vi "mean_Scope.vi"(0 "instrument handle in":refnum<k15>, 5 "pulses":i32, 7 "channels":string="0", 9 "record length":i32, 11 "error in":errorcluster) -> (4 "instrument handle out":refnum<k15>, 6 "signal out":dbl[](array[numeric]), 8 "dt":dbl, 15 "error out":errorcluster)   [LabVIEW 2016]
uses:
  <instrlib>/niScope/Acquire/niScope Read WDT.vi
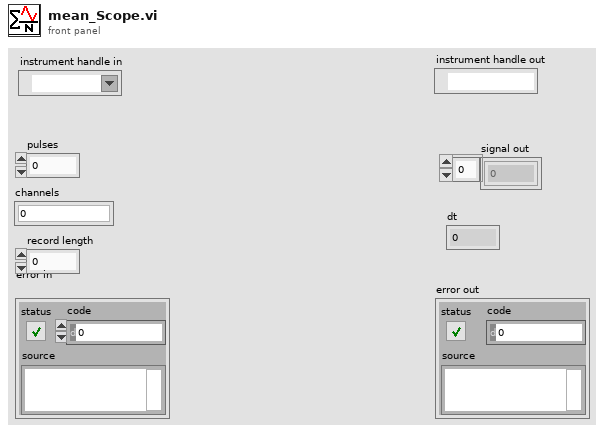
[diagram p1: front panel]
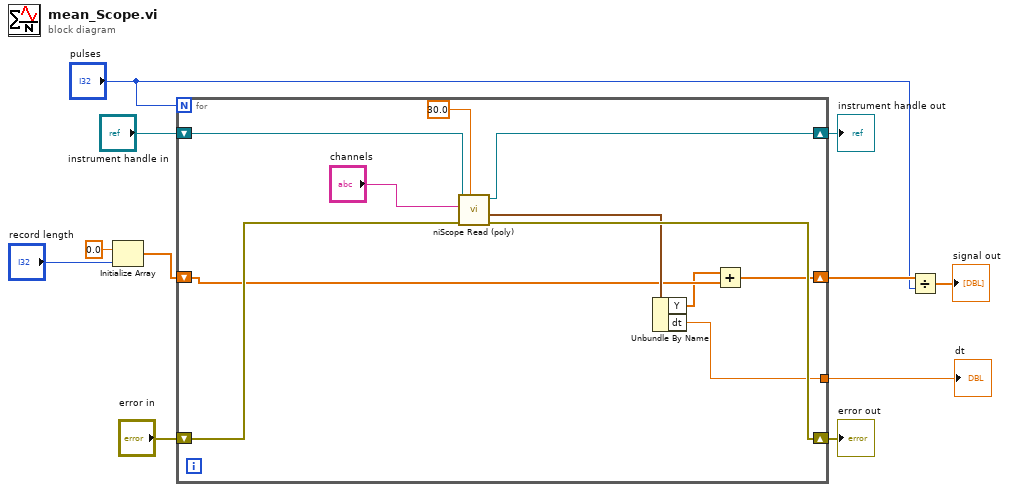
[diagram p0: block diagram]
diagram:
  n1 = Initialize Array(0.0 ("element"), "record length") -> (w8:dbl[])
  n2 = for {
    N: "pulses" -> [_]
    shift-right: [w18] -> w5
    shift-left: "error in" -> [w20]
    shift-right: [w19] -> w6
    shift-left: "instrument handle in" -> [w22]
    shift-right: [w15] -> w3
    shift-left: w8 -> [w16]
    tunnel: [w13] -> w4
    n3 = call-poly <instrlib>:"niScope Read (poly).vi"("timeout"=30.0, "error in"=w20, "channels"="channels", "instrument handle"=w22) -> ("error out"=w18:errorcluster, "wfm"=w17:waveform(dbl), "instrument handle out"=w19:refnum<k15>)  [unwired: 4 in, 1 out]
    n4 = Unbundle By Name(w17) -> ("Y"=w14:dbl[], "dt"=w13:dbl)
    n5 = Add(x=w14, y=w16) -> (x+y=w15:dbl[])
  }
  "instrument handle out" <- w6
  "error out" <- w5
  "dt" <- w4
  n6 = Divide(x=w3, y="pulses") -> (x/y=→"signal out":dbl[])
